vi "fgv_gmap.vi"() -> ()   [LabVIEW 2019]
panel:
  in  "cmd":enum16{""}(ring)
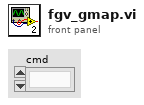
[diagram p1: front panel]
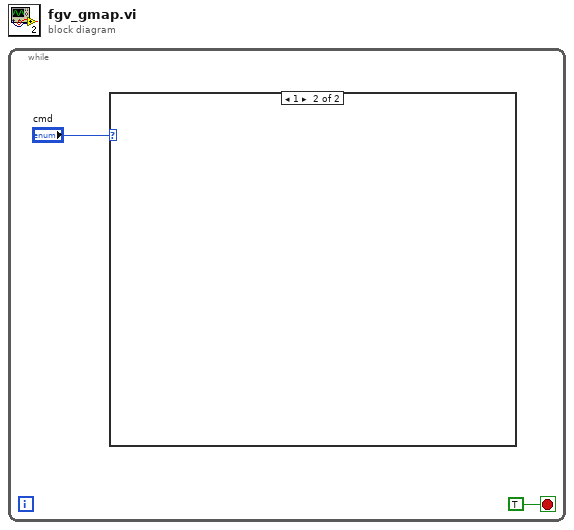
[diagram p0: block diagram]
diagram:
  n1 = while {
    stop <- TRUE stop-if-true
    n2 = case shown="\"1\"" "cmd" {
      frame "", Default {
      }
      frame 1 {
      }
    }
  }
